vi "Omni-teste-2.vi"() -> ()   [LabVIEW 2012]
panel:
  out "XY Graph 2":T1(graph)
  out "Waveform Graph":dbl[][](graph)
  in  "Medias":i32
  out "Length":i32
  out "x-y":u32
  in  "stop":bool
  in  "Integration Time":i32
  out "Number of Spectrometers":i32
  out "XY Graph":T1(graph)
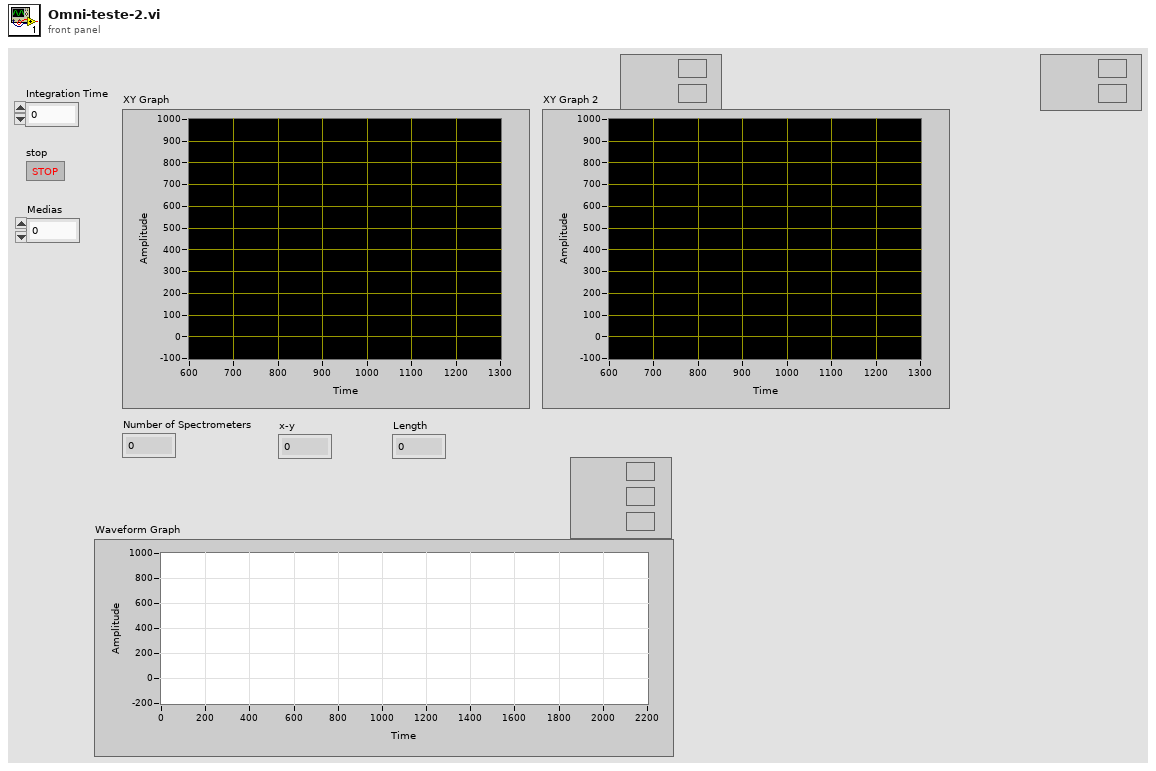
[diagram p1: front panel]
types:
  T1 = cluster{"WL Values":dbl[], "Spectrum Values":dbl[]}
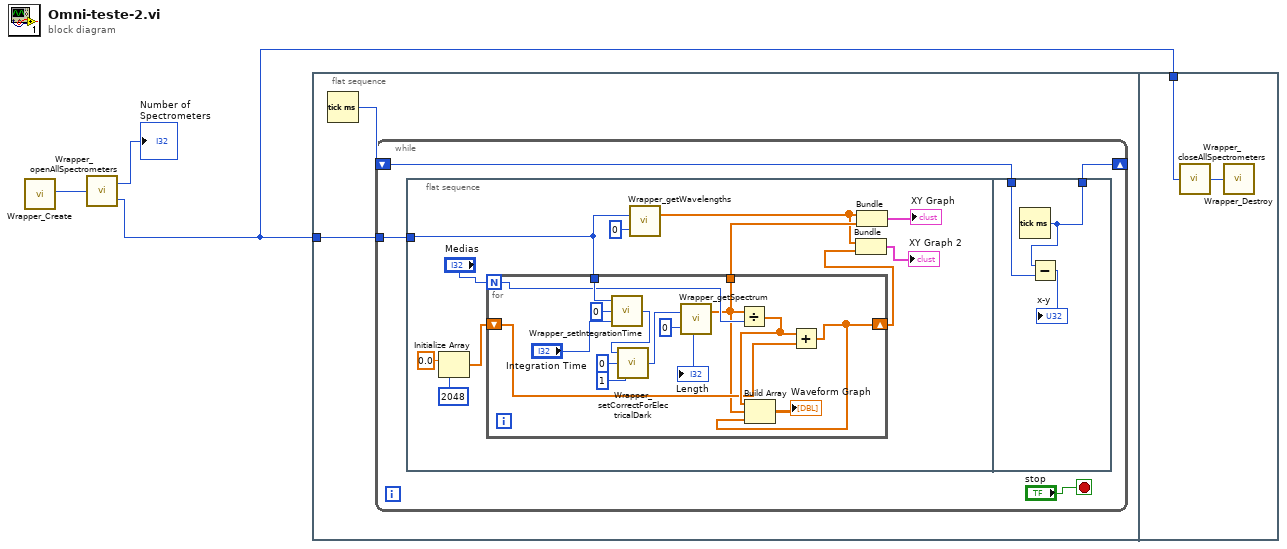
[diagram p0: block diagram]
diagram:
  n1 = call "Wrapper_Create.vi"() -> ("Wrapper"=w3:u32)
  n2 = call "Wrapper_openAllSpectrometers.vi"("Wrapper In"=w3) -> ("Number of Spectrometers"=→"Number of Spectrometers":i32, "Wrapper Out"=w1:u32)
  n3 = flat-sequence {
    tunnel: w1 -> [w5]
    tunnel: w1 -> [w40]
    frame #0 {
      n4 = Tick Count (ms)() -> (millisecond timer value=w4:u32)
      n5 = while {
        tunnel: w5 -> [w9]
        shift-right: [w6] -> _
        shift-left: w4 -> [w7]
        stop <- "stop" stop-if-true
        n6 = flat-sequence {
          tunnel: w9 -> [w11]
          tunnel: w7 -> [w38]
          tunnel: [w36] -> w6
          frame #0 {
            n7 = Initialize Array(0.0 ("element"), 2048 ("dimension size")) -> (w17:dbl[])
            n8 = for {
              N: "Medias" -> [w26]
              tunnel: w11 -> [w32]
              shift-right: [w22] -> w14
              shift-left: w17 -> [w23]
              tunnel: [w21] -> w16
              n9 = call "Wrapper_setIntegrationTime.vi"("Integration Time"="Integration Time", "Index"=0, "Wrapper In"=w32) -> ("Wrapper Out"=w30:u32)
              n10 = call "Wrapper_setCorrectForElectricalDark.vi"("On/Off"=1, "Index"=0, "Wrapper In"=w30) -> ("Wrapper Out"=w27:u32)
              n11 = call "Wrapper_getSpectrum.vi"("Index"=0, "Wrapper"=w27) -> ("Length"=→"Length":i32, "Spectrum Values"=w21:dbl[])
              n12 = Divide(x=w21, y=w26) -> (x/y=w24:dbl[])
              n13 = Add(x=w24, y=w23) -> (x+y=w22:dbl[])
              n14 = Build Array(w24, w21, w22) -> (→"Waveform Graph":dbl[][])
            }
            n15 = call "Wrapper_getWavelengths.vi"("Index"=0, "Wrapper"=w11) -> ("WL Values"=w10:dbl[])  [unwired: 1 out]
            n16 = Bundle("WL Values"=w10, w14) -> (→"XY Graph 2":cluster{"WL Values":dbl[], dbl[]})  [unwired: 1 in]
            n17 = Bundle("WL Values"=w10, "Spectrum Values"=w16) -> (→"XY Graph":T1)  [unwired: 1 in]
          }
          frame #1 {
            n18 = Tick Count (ms)() -> (millisecond timer value=w36:u32)
            n19 = Subtract(x=w36, y=w38) -> (x-y=→"x-y":u32)
          }
        }
      }
    }
    frame #1 {
      n20 = call "Wrapper_closeAllSpectrometers.vi"("Wrapper In"=w40) -> ("Wrapper Out"=w39:u32)
      n21 = call "Wrapper_Destroy.vi"("Wrapper"=w39) -> ()
    }
  }
